vi "Eurotherm - VISA Serial - Read Reply.vi"(0 "VISA resource name":refnum<visa-resource-name>, 2 "Read Reply":bool, 5 "Timeout (ms)":u32=5000, 11 "error in (no error)":errorcluster) -> (4 "dup VISA resource name":refnum<visa-resource-name>, 8 "read buffer":string, 10 "Success":bool, 15 "error out":errorcluster)   [LabVIEW 2011]
panel:
  out "bytes read":u32
  out "Iterations":i32
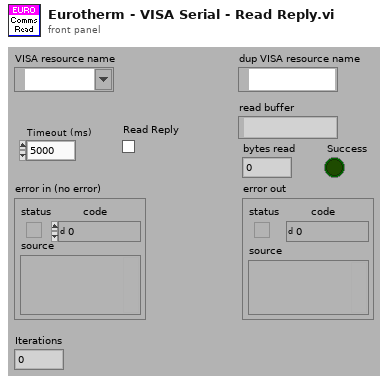
[diagram p1: front panel]
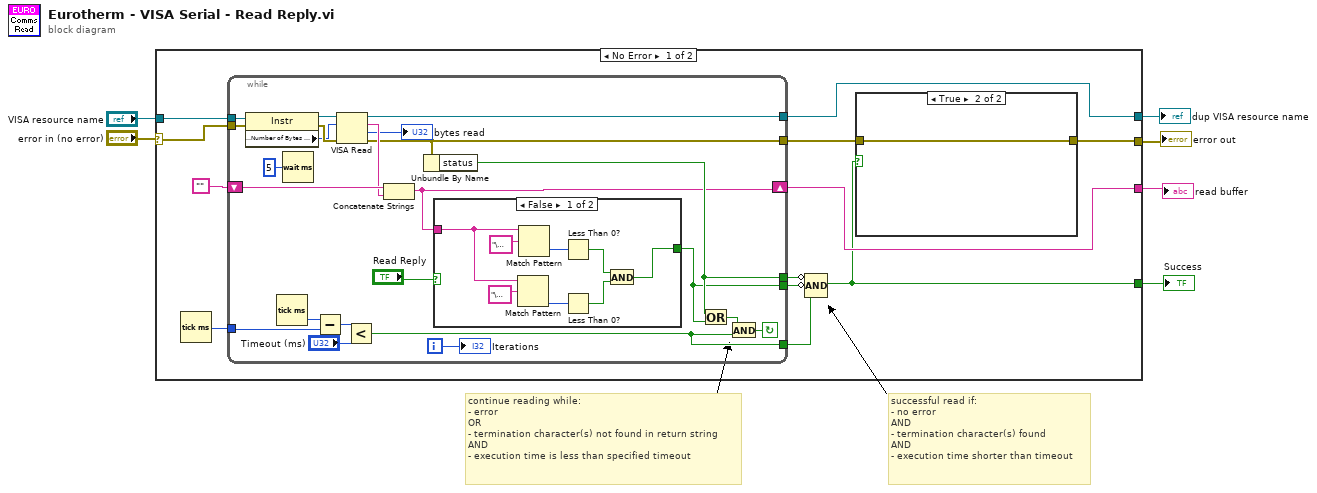
[diagram p0: block diagram]
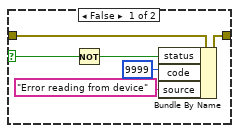
[diagram p2: hidden frame]
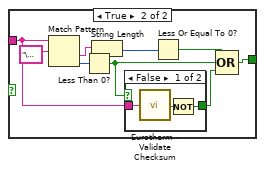
[diagram p3: hidden frame]
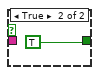
[diagram p4: hidden frame]
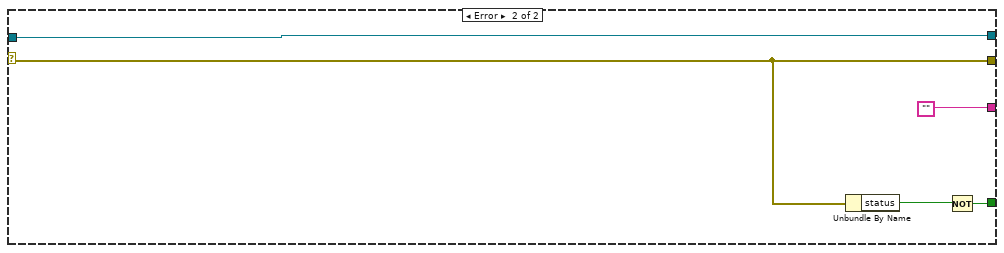
[diagram p5: hidden frame]
diagram:
  # "successful read if:\n- no error\nAND\n- termination character(s) found\nAND\n- execution time shorter than timeout"
  # "continue reading while:\n- error\nOR\n- termination character(s) not found in return string\nAND\n- execution time is less than specified timeout"
  n1 = case shown="No Error" "error in (no error)" {
    selector: "error in (no error)" -> [w17 w72]
    tunnel: [w9 w72] -> w1
    tunnel: "VISA resource name" -> [w18 w74]
    tunnel: [w11 w74] -> w4
    tunnel: [w8 ""] -> w3
    tunnel: [w7 w70] -> w2
    frame No Error {
      n2 = Tick Count (ms)() -> (millisecond timer value=w15:u32)
      n3 = while {
        tunnel: [w34] -> w10
        tunnel: [w48] -> w11
        tunnel: w18 -> [w47]
        tunnel: w17 -> [w45]
        shift-right: [w27] -> w8
        shift-left: "" -> [w43]
        tunnel: w15 -> [w37]
        tunnel: [w30] -> w14
        tunnel: [w28] -> w13
        tunnel: [w31] -> w12
        i -> [w39]
        stop <- w33 continue-if-true
        n4 = property class="Instr"(reference=w47, error in=w45) -> (reference out=w46:refnum<visa-resource-name>, error out=w44:errorcluster, "Serial Settings:Number of Bytes at Serial Port"=w26:u32)
        n5 = Tick Count (ms)() -> (millisecond timer value=w38:u32)
        n6 = Wait (ms)(milliseconds to wait=u32 5) -> ()  [unwired: 1 out]
        n7 = Subtract(x=w38, y=w37) -> (x-y=w36:u32)
        n8 = VISA Read(VISA resource name=w46, byte count=w26, error in (no error)=w44) -> (VISA resource name out=w48:refnum<visa-resource-name>, read buffer=w42:string, return count=→"bytes read":u32, error out=w34:errorcluster)
        n9 = Less?(x=w36, y="Timeout (ms)") -> (x < y?=w31:bool)
        n10 = Concatenate Strings(w43, w42) -> (w27:string)
        n11 = Unbundle By Name(w34) -> ("status"=w30:bool)
        n12 = case shown="False" "Read Reply" {
          tunnel: w27 -> [w53 w59]
          tunnel: [w49 w60] -> w28
          frame False {
            n13 = Match Pattern(string=w53, regular expression="\u0015") -> (offset past match=w52:i32)  [unwired: 1 in, 3 out]
            n14 = Match Pattern(string=w53, regular expression="\u0006") -> (offset past match=w56:i32)  [unwired: 1 in, 3 out]
            n15 = Less Than 0?(x=w56) -> (x < 0?=w51:bool)
            n16 = Less Than 0?(x=w52) -> (x < 0?=w50:bool)
            n17 = And(x=w51, y=w50) -> (x .and. y?=w49:bool)
          }
          frame True {
            n18 = Match Pattern(string=w59, regular expression="\u0003") -> (after substring=w61:string, offset past match=w64:i32)  [unwired: 1 in, 2 out]
            n19 = Less Than 0?(x=w64) -> (x < 0?=w58:bool)
            n20 = String Length(string=w61) -> (length=w63:i32)
            n21 = case shown="False" w58 {
              tunnel: w59 -> [w68 _]
              tunnel: [w66 TRUE] -> w57
              frame False {
                n22 = call "Eurotherm - Validate Checksum.vi"("Reply"=w68) -> ("Checksum Valid"=w67:bool)  [unwired: 14 in]
                n23 = Not(x=w67) -> (.not. x?=w66:bool)
              }
              frame True {
              }
            }
            n24 = Less Or Equal To 0?(x=w63) -> (x <= 0?=w62:bool)
            n25 = Compound Arithmetic op=OR(w62, w58, w57) -> (w60:bool)
          }
        }
        n26 = Or(x=w30, y=w28) -> (x .or. y?=w32:bool)
        n27 = And(x=w32, y=w31) -> (x .and. y?=w33:bool)
        "Iterations" <- w39
      }
      n28 = Compound Arithmetic op=AND(invert w14, invert w13, w12) -> (w7:bool)
      n29 = case shown="True" w7 {
        selector: w7 -> [w21 _]
        tunnel: w10 -> [w24 w25]
        tunnel: [w23 w25] -> w9
        frame False {
          n30 = Not(x=w21) -> (.not. x?=w22:bool)
          n31 = Bundle By Name(cluster=w24, "status"=w22, "code"=9999, "source"="Error reading from device") -> (w23:errorcluster)
        }
        frame True {
        }
      }
    }
    frame Error {
      n32 = Unbundle By Name(w72) -> ("status"=w71:bool)
      n33 = Not(x=w71) -> (.not. x?=w70:bool)
    }
  }
  "error out" <- w1
  "dup VISA resource name" <- w4
  "read buffer" <- w3
  "Success" <- w2
